vi "OAT Orbit Locate Waveform Segment.vi"(8 "tach cycle(1)":i32=1, 9 "orbit segment":cluster{"position":dbl, "tach duty":dbl} {"tach duty" format="%.2f"; "position" format="%.2f"}, 10 "pulse/revolution (1)":i32=1, 11 "speed profile":T1 {"speed [RPM]" format="%.2f"; "time [s]" format="%.2f"}) -> (1 "instant RPM":dbl format="%.2f", 2 "duration":dbl format="%.2e", 3 "start points":dbl[](array[numeric]) format="%.2f")   [LabVIEW 2017]
uses:
  <vilib>/addons/Sound and Vibration/Order Analysis/Tach Process/SubVIs/speed profile.ctl
  <vilib>/Analysis/2dsp.llb/Decimate (single shot, DBL).vi
  <vilib>/Analysis/NI_AALPro.lvlib
  <vilib>/addons/Sound and Vibration/Order Analysis/Tach Process/SoundVib_TachProcess.lvlib
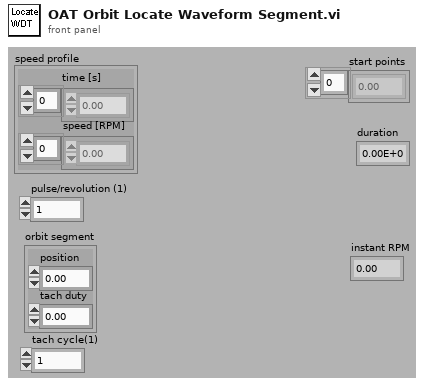
[diagram p1: front panel]
types:
  T1 = typedef "SoundVib_TachProcess.lvlib/speed profile.ctl" = cluster{"time [s]":dbl[], "speed [RPM]":dbl[]}
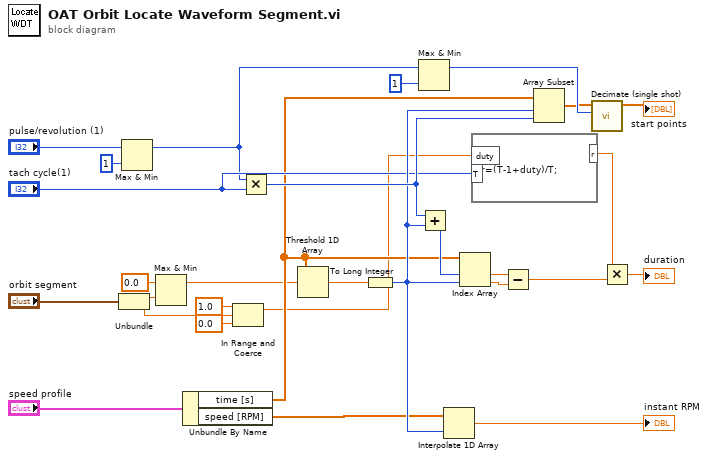
[diagram p0: block diagram]
diagram:
  n1 = Unbundle("orbit segment") -> ("position"=w15:dbl, "tach duty"=w12:dbl)
  n2 = Max & Min(x="pulse/revolution (1)", y=1) -> (max(x,y)=w2:i32)  [unwired: 1 out]
  n3 = Max & Min(x=0.0 ("y"), y=w15) -> (max(x,y)=w13:dbl)  [unwired: 1 out]
  n4 = Unbundle By Name("speed profile") -> ("time [s]"=w22:dbl[], "speed [RPM]"=w21:dbl[])
  n5 = In Range and Coerce(upper limit=1.0, x=w12, lower limit=0.0) -> (coerced(x)=w10:dbl)  [unwired: 1 out]
  n6 = Multiply(x=w2, y="tach cycle(1)") -> (x*y=w29:i32)
  n7 = Threshold 1D Array(2:w13, 3:w22) -> (0:w16:dbl)  [unwired: 1 in]
  n8 = To Long Integer(number=w16) -> (32bit integer=w27:i32)
  n9 = Max & Min(x=w2, y=1) -> (max(x,y)=w19:i32)  [unwired: 1 out]
  n10 = Add(x=w29, y=w27) -> (x+y=w28:i32)
  n11 = Interpolate 1D Array(1:w27, 2:w21) -> (0:→"instant RPM":dbl)
  n12 = Index Array(array=w22, index #1=w28, index #2=w27) -> (element #1=w4:dbl, element #2=w3:dbl)
  n13 = formula code="r=(T-1+duty)/T;"("duty"=w10, "T"="tach cycle(1)") -> ("r"=w23:dbl)
  n14 = Subtract(x=w4, y=w3) -> (x-y=w17:dbl)
  n15 = Array Subset(array=w22, index=w27, length=w29) -> (w18:dbl[])
  n16 = call-poly <vilib>:"Decimate (single shot).vi"("decimating factor"=w19, "X"=w18) -> ("Decimated Array"=→"start points":dbl[])  [unwired: 8 in, 1 out]
  n17 = Multiply(x=w23, y=w17) -> (x*y=→"duration":dbl)
